vi "DEL.vi"(0 "System no.":i32=1 min=1 max=4 step=1, 3 "Delay time":dbl=1.0 min=0.0 max=20.0 step=1.0, 5 "error in":errorcluster) -> (19 "error out":errorcluster)   [LabVIEW 2020]
doc: "Delays the command interpreter of specified system for given\n\"Delay time\". DEL is used within macros primarily. Do not mistace MAC DEL which deletes macros for DEL which delays.\n\nAll systems: Delay time unit is ms.\n\nE-816: This command cannot be issued to a slave. Check controller manual to find out if DEL is supported.\n\nC-887, F-206, M-8X0: Only for GCS syntax version = GCS 2.0 or higher (check with CSV?.vi. If CSV?.vi is not supported, syntax version is GCS 1.0)."
panel:
  # "Delays the command interpreter of specified system for given\n\"Delay time\". DEL is used within macros primarily."
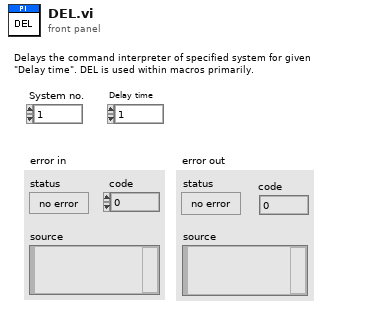
[diagram p1: front panel]
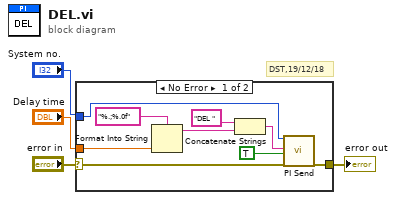
[diagram p0: block diagram]
diagram:
  # "DST,19/12/18"
  n1 = case shown="No Error" "error in" {
    selector: "error in" -> [w5 w14]
    tunnel: "System no." -> [w11 _]
    tunnel: "Delay time" -> [w8 _]
    tunnel: [w6 w14] -> w2
    frame No Error {
      n2 = Format Into String(format string="%.;%.0f" ("Format String"), w8) -> (resulting string=w7:string)  [unwired: 2 in, 1 out]
      n3 = Concatenate Strings("DEL ", w7) -> (w10:string)
      n4 = call "PI Send.vi"("System no."=w11, "String to send"=w10, "Attach termination char.?"=TRUE ("Attach Linefeed?"), "error in"=w5) -> ("error out"=w6:errorcluster)  [unwired: 2 in, 13 out]
    }
    frame Error {
    }
  }
  "error out" <- w2
